vi "WaitLimits.vi"() -> ()   [LabVIEW 2015]
panel:
  out "Wait_Time":i32
  in  "Max_Time":i32=500
  in  "Min_Time":i32=10
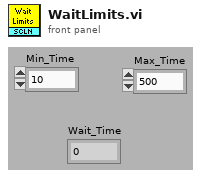
[diagram p1: front panel]
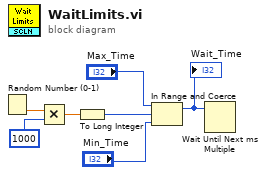
[diagram p0: block diagram]
diagram:
  n1 = Random Number (0-1)() -> (number: 0 to 1=w7:dbl)
  n2 = Multiply(x=w7, y=1000) -> (x*y=w6:dbl)
  n3 = To Long Integer(number=w6) -> (32bit integer=w4:i32)
  n4 = In Range and Coerce(upper limit="Max_Time", x=w4, lower limit="Min_Time") -> (coerced(x)=w1:i32)  [unwired: 1 out]
  "Wait_Time" <- w1
  n5 = Wait Until Next ms Multiple(millisecond multiple=w1) -> ()  [unwired: 1 out]
